vi "adjustTabControl.vi"(8 "error in (no error)":errorcluster, 11 "BaseSetting in":refnum<class "Setting.lvclass">) -> (0 "error out":errorcluster, 3 "BaseSetting out":refnum<class "Setting.lvclass">)   [LabVIEW 2016, in "Setting.lvclass"]
uses:
  Setting.lvclass
  Setting.lvclass/Setting.ctl
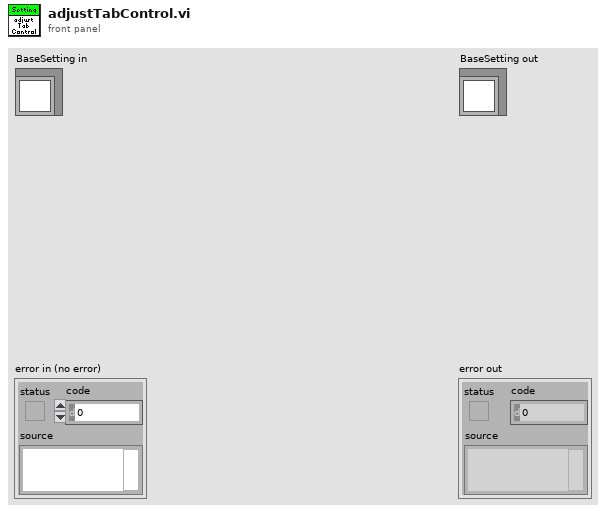
[diagram p1: front panel]
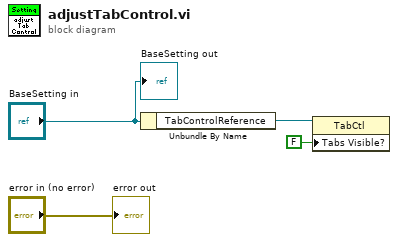
[diagram p0: block diagram]
diagram:
  n1 = Unbundle By Name("BaseSetting in") -> ("TabControlReference"=w4:refnum<vi>)
  n2 = property class="TabCtl"(reference=w4, "Tabs Visible?"=FALSE) -> ()  [unwired: 1 in, 2 out]
  "error out" <- "error in (no error)"
  "BaseSetting out" <- "BaseSetting in"
